vi "Stop Core.vi"(10 "final error code":i32, 11 "Customer With Cell Phone in":refnum<class "Customer With Cell Phone.lvclass">) -> (3 "Customer With Cell Phone out":refnum<class "Customer With Cell Phone.lvclass">)   [LabVIEW 2023, in "Customer With Cell Phone.lvlib" / "Customer With Cell Phone.lvclass"]
doc: "(<B>Filename</B>: Actor Framework.lvlib:Actor.lvclass:Stop Core.vi)\n\nDefines what the actor does before it stops. Use the <B>final error code</B> input to determine whether the actor shut down in response to an error.\n\nBy default, this method does nothing. A descendant class may override it to define behavior, such as shutting down any processes the actor initiated in its override of the Actor Core method."
uses:
  Customer With Cell Phone.lvclass
  Customer With Cell Phone.lvclass/Customer With Cell Phone.ctl
  Customer.lvclass
panel:
  out "error out":errorcluster
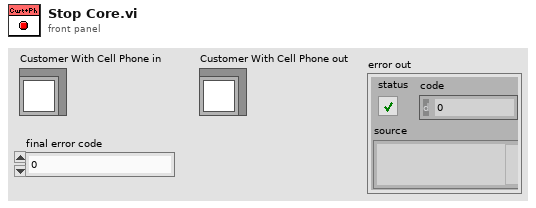
[diagram p1: front panel]
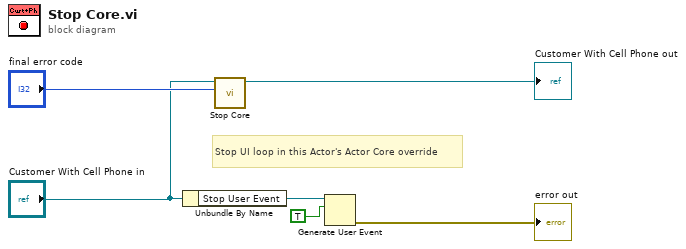
[diagram p0: block diagram]
diagram:
  # "Stop UI loop in this Actor's Actor Core override"
  n1 = Unbundle By Name("Customer With Cell Phone in") -> ("Stop User Event"=w3:refnum<user-event>)
  n2 = call-parent "Stop Core.vi"("final error code"="final error code", "Customer in"="Customer With Cell Phone in") -> ("Customer out"=→"Customer With Cell Phone out":refnum<class "Customer With Cell Phone.lvclass">)  [unwired: 9 in]
  n3 = Generate User Event(user event=w3, event data cluster=TRUE ("event data")) -> (error out=→"error out":errorcluster)  [unwired: 2 in, 1 out]
